vi "FGV Betriebsstundenzaehler.vi"(6 "BSZ Aktionen":T1=enum."Initialisieren", 9 "Betriebsstunden FT-IR":dbl, 11 "Betriebsstunden Pumpe":dbl) -> (1 "Betriebsstunden FT-IR":dbl format="%#_15g", 3 "Betriebsstunden Pumpe":dbl format="%#_15g")   [LabVIEW 2020, in "Betriebsstundenzaehler.lvlib"]
uses:
  Betriebsstundenzaehler.lvlib
  FGV BSZ Aktionen.ctl
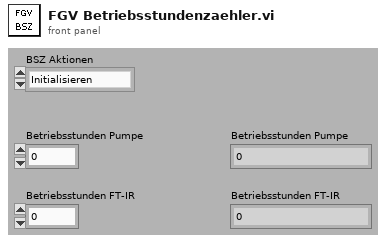
[diagram p1: front panel]
types:
  T1 = typedef "Betriebsstundenzaehler.lvlib/FGV BSZ Aktionen.ctl" = enum16{"Lesen", "Initialisieren", "Starten Pumpe", "Zählen Pumpe", "Starten FT-IR", "Zählen FT-IR"}
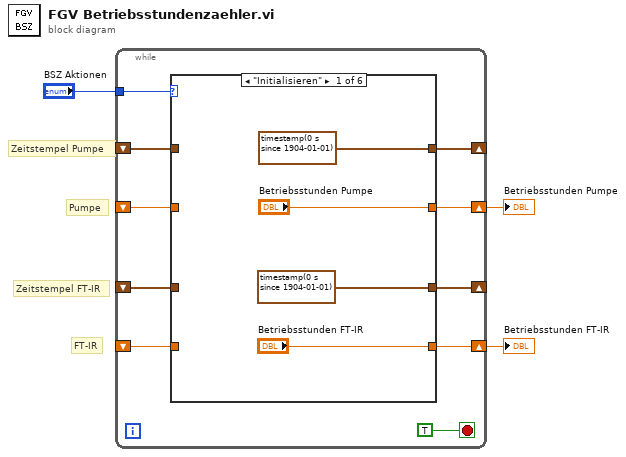
[diagram p0: block diagram]
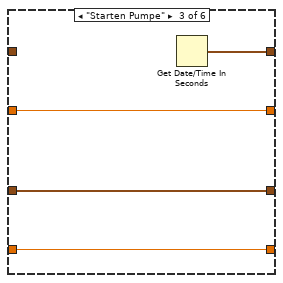
[diagram p3: hidden frame]
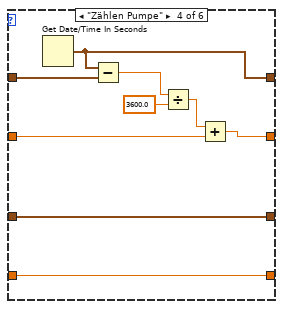
[diagram p4: hidden frame]
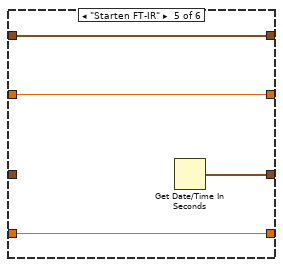
[diagram p5: hidden frame]
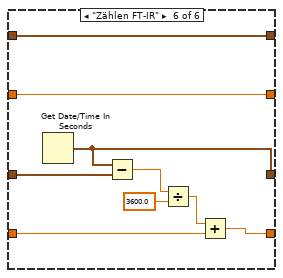
[diagram p6: hidden frame]
diagram:
  # "FT-IR"
  # "Pumpe"
  # "Zeitstempel FT-IR"
  # "Zeitstempel Pumpe"
  n1 = while {
    shift-right: [w11] -> w2
    shift-left: _ -> [w12]
    tunnel: "BSZ Aktionen" -> [w13]
    shift-right: [w10] -> _
    shift-left: _ -> [w9]
    shift-right: [w7] -> _
    shift-left: _ -> [w5]
    shift-right: [w6] -> w1
    shift-left: _ -> [w4]
    stop <- TRUE stop-if-true
    n2 = case shown="\"Initialisieren\"" w13 {
      tunnel: w12 -> [_ w21 w25 w32 w38 w39]
      tunnel: ["Betriebsstunden Pumpe" w21 w25 w31 w38 w39] -> w11
      tunnel: [timestamp(0 s since 1904-01-01) w20 w24 w30 w36 w40] -> w10
      tunnel: w9 -> [_ w20 _ w29 w36 w40]
      tunnel: [timestamp(0 s since 1904-01-01) w19 w23 w27 w35 w44] -> w7
      tunnel: ["Betriebsstunden FT-IR" w18 w22 w26 w37 w42] -> w6
      tunnel: w5 -> [_ w19 w23 w27 _ w41]
      tunnel: w4 -> [_ w18 w22 w26 w37 w43]
      frame "Initialisieren" {
      }
      frame "Lesen", Default {
      }
      frame "Starten Pumpe" {
        n3 = Get Date/Time In Seconds() -> (seconds since 1Jan1904=w24:timestamp)
      }
      frame "Zählen Pumpe" {
        n4 = Get Date/Time In Seconds() -> (seconds since 1Jan1904=w30:timestamp)
        n5 = Subtract(x=w30, y=w29) -> (x-y=w28:dbl)
        n6 = Divide(x=w28, y=3600.0) -> (x/y=w33:dbl)
        n7 = Add(x=w33, y=w32) -> (x+y=w31:dbl)
      }
      frame "Starten FT-IR" {
        n8 = Get Date/Time In Seconds() -> (seconds since 1Jan1904=w35:timestamp)
      }
      frame "Zählen FT-IR" {
        n9 = Get Date/Time In Seconds() -> (seconds since 1Jan1904=w44:timestamp)
        n10 = Subtract(x=w44, y=w41) -> (x-y=w45:dbl)
        n11 = Divide(x=w45, y=3600.0) -> (x/y=w46:dbl)
        n12 = Add(x=w46, y=w43) -> (x+y=w42:dbl)
      }
    }
  }
  "Betriebsstunden Pumpe" <- w2
  "Betriebsstunden FT-IR" <- w1
